vi "Z-axis PID feedback loop (SubVI).vi"(0 "current amp.":dbl, 1 "ms to wait for PID":u32=50, 3 "output range":cluster{"output high":dbl, "output low":dbl}={"output high"=11.0, "output low"=9.0} {"output low" format="%.2f"; "output high" format="%.2f"}, 5 "set amp.":dbl, 9 "manual set amp.":dbl, 11 "PID gains":T1={"proportional gain (Kc)"=0.1, "integral time (Ti, min)"=1.0, "derivative time (Td, min)"=0.0} {"derivative time (Td, min)" format="%.3f"; "integral time (Ti, min)" format="%.3f"; "proportional gain (Kc)" format="%.3f"}, 12 "manual set?":bool, 13 "T=feedback; F=not":bool, 14 "Polyfit Coeff. \n(amp. to position)":dbl[](array[numeric])) -> (4 "z position before move\nor no feedback=z drift (um)":dbl, 6 "z position of PID target (um)":dbl, 15 "z position after moved (um)":dbl)   [LabVIEW 2014]
uses:
  <vilib>/Analysis/polynomials.llb/Scalar Polynomial Evaluation (DBL).vi
  <vilib>/addons/control/pid/pid.llb/PID (DBL).vi
  Main-Stage-PI/(Global) Current handle and LaserPower_YCC.vi
  <vilib>/addons/control/pid/NI_PID_pid.lvlib
  <vilib>/Analysis/NI_AALPro.lvlib
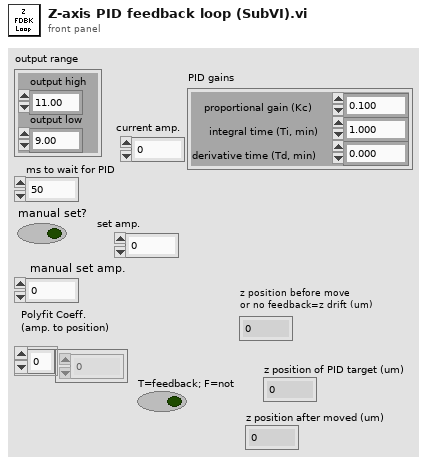
[diagram p1: front panel]
types:
  T1 = cluster{"proportional gain (Kc)":dbl, "integral time (Ti, min)":dbl, "derivative time (Td, min)":dbl}
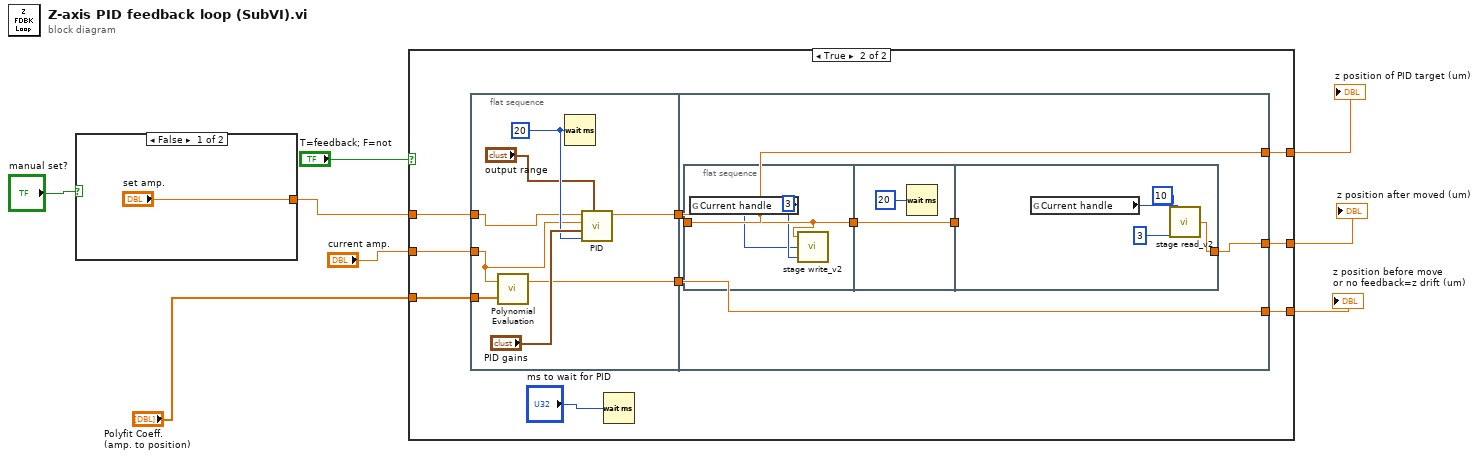
[diagram p0: block diagram]
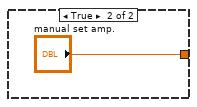
[diagram p2: hidden frame]
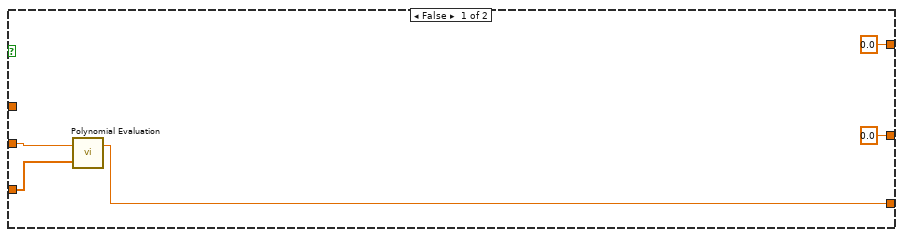
[diagram p3: hidden frame]
diagram:
  n1 = case shown="False" "manual set?" {
    tunnel: ["set amp." "manual set amp."] -> w8
    frame False {
    }
    frame True {
    }
  }
  n2 = case shown="True" "T=feedback; F=not" {
    tunnel: w8 -> [_ w24]
    tunnel: "current amp." -> [w15 w23]
    tunnel: [0.0 ("Position out") w22] -> w6
    tunnel: [0.0 ("output") w21] -> w5
    tunnel: [w13 w20] -> w4
    tunnel: "Polyfit Coeff. \n(amp. to position)" -> [w14 w19]
    frame False {
      n3 = call-poly <vilib>:"Polynomial Evaluation.vi"("P(x)"=w14, "a"=w15) -> ("P(a)"=w13:dbl)  [unwired: 1 out]
    }
    frame True {
      n4 = flat-sequence {
        tunnel: w24 -> [w25]
        tunnel: w23 -> [w27]
        tunnel: [w31] -> w18
        tunnel: [w30] -> w17
        tunnel: w19 -> [w26]
        tunnel: w18 -> [w36]
        tunnel: [w37] -> w22
        tunnel: [w36] -> w21
        tunnel: [w35] -> w20
        tunnel: w17 -> [w35]
        frame #0 {
          w29 = u32 20 ("milliseconds to wait")
          n5 = call-poly <vilib>:"Polynomial Evaluation.vi"("P(x)"=w26, "a"=w27) -> ("P(a)"=w30:dbl)  [unwired: 1 out]
          n6 = Wait (ms)(milliseconds to wait=w29) -> ()  [unwired: 1 out]
          n7 = call-poly <vilib>:"PID.vi"("output range"="output range", "dt (s)"=w29, "PID gains"="PID gains", "process variable"=w27, "setpoint"=w25) -> ("output"=w31:dbl)  [unwired: 5 in, 1 out]
        }
        frame #1 {
          n8 = flat-sequence {
            tunnel: w36 -> [w40]
            tunnel: [w40] -> w34
            tunnel: [w41] -> w33
            tunnel: w34 -> [w41]
            tunnel: [w43] -> w37
            tunnel: w33 -> [_]
            frame #0 {
              n9 = global read "(Global) Current handle and LaserPower_YCC.vi" "Current handle"() -> (w38:i32)
              n10 = call "stage write_v2.vi"("axis"=u32 3 ("Axis (X1,Y2,Z3)"), "Incoming Handle"=w38, "position"=w40) -> ()  [unwired: 2 in, 1 out]
            }
            frame #1 {
              n11 = Wait (ms)(milliseconds to wait=u32 20) -> ()  [unwired: 1 out]
            }
            frame #2 {
              n12 = global read "(Global) Current handle and LaserPower_YCC.vi" "Current handle"() -> (w45:i32)
              n13 = call "stage read_v2.vi"("Axis"=u32 3 ("axis"), "Incoming Handle"=w45, "read #"=10) -> ("position (um)"=w43:dbl)  [unwired: 1 in, 1 out]
            }
          }
        }
      }
      n14 = Wait (ms)(milliseconds to wait="ms to wait for PID") -> ()  [unwired: 1 out]
    }
  }
  "z position of PID target (um)" <- w5
  "z position after moved (um)" <- w6
  "z position before move\nor no feedback=z drift (um)" <- w4
